vi "Assert 32 bit or less wired to I64 bit Type.vi"   [LabVIEW 2017]
uses:
  eca23347-5497-43b4-94af-ed5bf14f2a90.vi
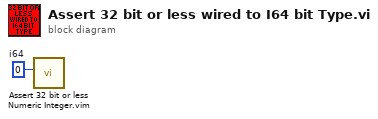
[diagram p0: block diagram]
diagram:
  w1 = i64 0  # i64
  n1 = call "Assert 32 bit or less Numeric Integer.vim"("Item in"=w1) -> ()  [unwired: 10 in, 1 out]
